vi "Agilent PWM Set Offset Status.vi"(7 "Agilent PWM":T1, 8 "error in (no error)":errorcluster, 10 "On/Off":bool, 11 "VISA Resource Name":refnum<visa-resource-name>) -> (0 "error out":errorcluster, 3 "dup VISA Resource Name":refnum<visa-resource-name>)   [LabVIEW 2011]
doc: "This VI for the HP 8753 is used to read the sweep type.\n\n0 LINEAR FREQ\n1 LOG FREQ\n2 LIST FREQ\n3 CW TIME\n4 POWER SWEEP"
uses:
  TypeDefs/Agilent PWM Instrument Info.ctl
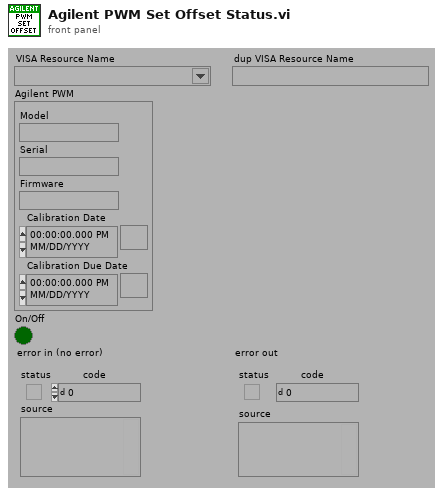
[diagram p1: front panel]
types:
  T1 = typedef "Agilent PWM Instrument Info.ctl" = cluster{"Model":string, "Serial":string, "Firmware":string, "Calibration Date":timestamp, "Calibration Due Date":timestamp}
  T2 = typedef "Agilent PWM Model.ctl" = enum16{"Not Supported", "E4418X", "E4419X", "U2000X"}
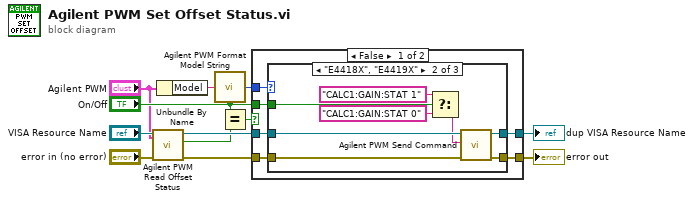
[diagram p0: block diagram]
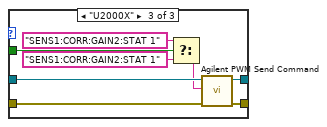
[diagram p3: hidden frame]
diagram:
  n1 = call "Agilent PWM Read Offset Status.vi"("Agilent PWM"="Agilent PWM", "error in (no error)"="error in (no error)", "VISA Resource Name"="VISA Resource Name") -> ("error out"=w7:errorcluster, "On/Off"=w6:bool, "dup VISA Resource Name"=w9:refnum<visa-resource-name>)  [unwired: 6 out]
  n2 = Unbundle By Name("Agilent PWM") -> ("Model"=w3:string)
  n3 = call "Agilent PWM Format Model String.vi"("Model"=w3) -> ("Model"=w1:T2)
  n4 = Equal?(x="On/Off", y=w6) -> (x = y?=w5:bool)
  n5 = case shown="False" w5 {
    tunnel: [w18 w38] -> w12
    tunnel: [w17 w37] -> w11
    tunnel: w9 -> [w16 w38]
    tunnel: w7 -> [w15 w37]
    tunnel: "On/Off" -> [w14 _]
    tunnel: w1 -> [w13 _]
    frame False {
      n6 = case shown="\"E4418X\", \"E4419X\"" w13 {
        tunnel: [w20 w28 w36] -> w18
        tunnel: [w19 w27 w35] -> w17
        tunnel: w16 -> [w20 w26 w34]
        tunnel: w15 -> [w19 w25 w33]
        tunnel: w14 -> [_ w24 w32]
        frame "Not Supported" {
        }
        frame "E4418X", "E4419X" {
          n7 = Select(t="CALC1:GAIN:STAT 1" ("write buffer"), s=w24, f="CALC1:GAIN:STAT 0" ("write buffer")) -> (s? t:f=w21:string)
          n8 = call "Agilent PWM Send Command.vi"("error in (no error)"=w25, "Command"=w21, "VISA Resource Name"=w26) -> ("error out"=w27:errorcluster, "dup VISA Resource Name"=w28:refnum<visa-resource-name>)  [unwired: 2 in, 5 out]
        }
        frame "U2000X" {
          n9 = Select(t="SENS1:CORR:GAIN2:STAT 1" ("write buffer"), s=w32, f="SENS1:CORR:GAIN2:STAT 1" ("write buffer")) -> (s? t:f=w29:string)
          n10 = call "Agilent PWM Send Command.vi"("error in (no error)"=w33, "Command"=w29, "VISA Resource Name"=w34) -> ("error out"=w35:errorcluster, "dup VISA Resource Name"=w36:refnum<visa-resource-name>)  [unwired: 2 in, 5 out]
        }
      }
    }
    frame True {
    }
  }
  "dup VISA Resource Name" <- w12
  "error out" <- w11
